vi "Init.vi"(8 "error in (no error)":errorcluster, 9 "SA Pin":string, 10 "Measurement Name":string) -> (0 "error out":errorcluster, 3 "LTE_ModAcc out":refnum<class "LTE_ModAcc.lvclass">)   [LabVIEW 2016, in "SeqAuto Evaluations.lvlib" / "LTE_ModAcc.lvclass"]
uses:
  LTE_ModAcc.lvclass
  C:/Sequence Automation/Plugins/SeqAuto IEvaluation.lvlibp/SeqAuto IEvaluation.lvclass
  LTE_ModAcc.lvclass/LTE_ModAcc.ctl
  Write SA Pin.vi
  Plugins/SeqAuto IEvaluation.lvlibp/Write Measurement Name.vi
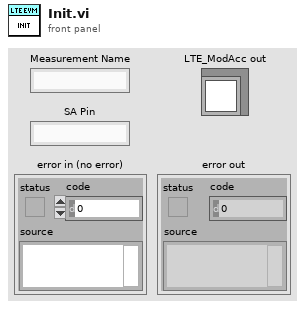
[diagram p1: front panel]
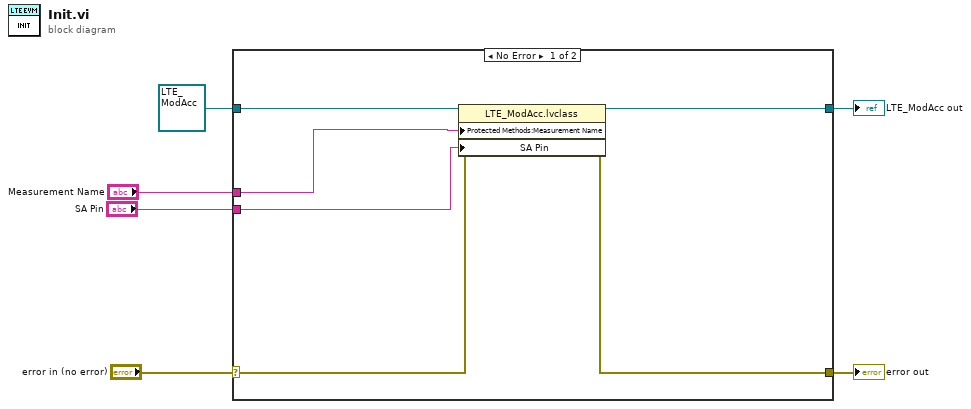
[diagram p0: block diagram]
diagram:
  n1 = case shown="No Error" "error in (no error)" {
    selector: "error in (no error)" -> [w12 w14]
    tunnel: [w11 w14] -> w5
    tunnel: [w9 w13] -> w3
    tunnel: refnum<class "LTE_ModAcc.lvclass"> refnum ("LTE_ModAcc in") -> [w10 w13]
    tunnel: "Measurement Name" -> [w8 _]
    tunnel: "SA Pin" -> [w7 _]
    frame No Error {
      n2 = property class="LTE_ModAcc.lvclass"(reference=w10, error in=w12, "Protected Methods:Measurement Name"=w8, "SA Pin"=w7) -> (reference out=w9:refnum<class "LTE_ModAcc.lvclass">, error out=w11:errorcluster)
    }
    frame Error {
    }
  }
  "error out" <- w5
  "LTE_ModAcc out" <- w3
